vi "4. Event-Driven State Machine - Traffic Light Simulator.vi"() -> ()   [LabVIEW 2018]
uses:
  Typedefs/States for Event-Driven State Machine.ctl
panel:
  in  "stop":bool
  in  "Press Green":bool
  in  "Press Yellow":bool
  in  "Press Red":bool
  out "Yellow":bool
  out "Green":bool
  out "Red":bool
  out "Traffic Lights Picture":picture
  # "Traffic Light Graphic Vector by Vecteezy\n(https://www.vecteezy.com/free-vector/graphic)"
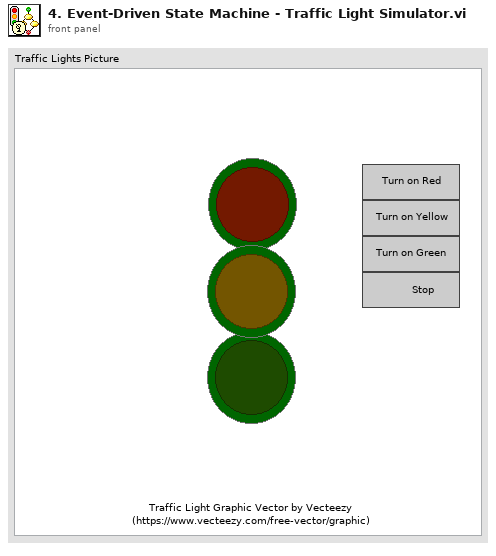
[diagram p1: front panel]
types:
  T1 = typedef "States for Event-Driven State Machine.ctl" = enum16{"Initialize", "Red", "Yellow", "Green", "Wait for Event", "Stop"}
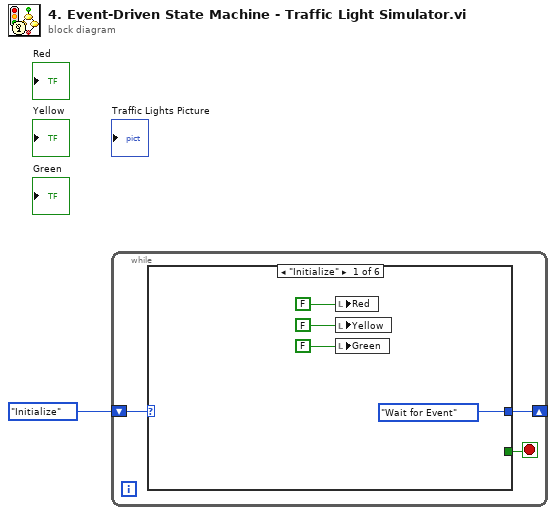
[diagram p0: block diagram]
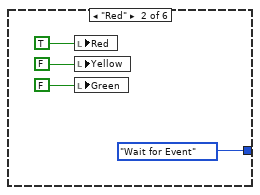
[diagram p2: hidden frame]
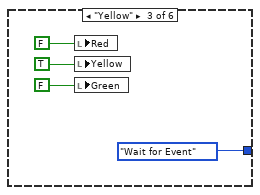
[diagram p3: hidden frame]
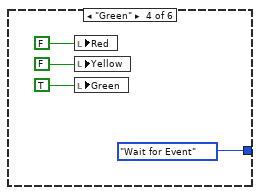
[diagram p4: hidden frame]
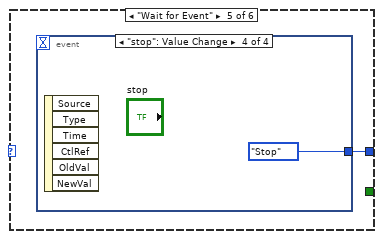
[diagram p5: hidden frame]
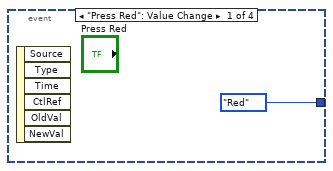
[diagram p6: hidden frame]
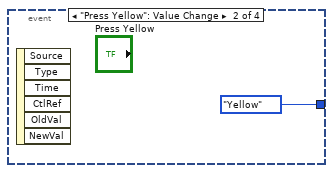
[diagram p7: hidden frame]
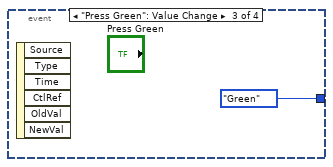
[diagram p8: hidden frame]
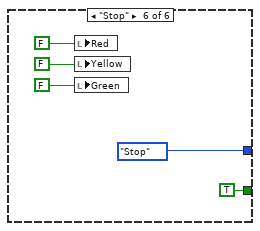
[diagram p9: hidden frame]
diagram:
  n1 = while {
    shift-right: [w3] -> _
    shift-left: States_for_Event-Driven_State_Machine."Initialize" -> [w4]
    stop <- w2 stop-if-true
    n2 = case shown="\"Initialize\"" w4 {
      tunnel: [States_for_Event-Driven_State_Machine."Wait for Event" States_for_Event-Driven_State_Machine."Wait for Event" States_for_Event-Driven_State_Machine."Wait for Event" States_for_Event-Driven_State_Machine."Wait for Event" w21 States_for_Event-Driven_State_Machine."Stop"] -> w3
      tunnel: [_ _ _ _ _ TRUE] -> w2
      frame "Initialize" {
        n3 = local write "Red"(FALSE ("Red")) -> ()
        n4 = local write "Yellow"(FALSE ("Red")) -> ()
        n5 = local write "Green"(FALSE ("Red")) -> ()
      }
      frame "Red" {
        n6 = local write "Red"(TRUE ("Red")) -> ()
        n7 = local write "Yellow"(FALSE ("Red")) -> ()
        n8 = local write "Green"(FALSE ("Red")) -> ()
      }
      frame "Yellow" {
        n9 = local write "Red"(FALSE ("Red")) -> ()
        n10 = local write "Yellow"(TRUE ("Red")) -> ()
        n11 = local write "Green"(FALSE ("Red")) -> ()
      }
      frame "Green" {
        n12 = local write "Red"(FALSE ("Red")) -> ()
        n13 = local write "Yellow"(FALSE ("Red")) -> ()
        n14 = local write "Green"(TRUE ("Red")) -> ()
      }
      frame "Wait for Event" {
        n15 = event shown="[3] \"stop\": Value Change" {
          selector: _ -> [_ _ _ _]
          dyn-events: _ -> [_ _ _ _]
          timeout: _ -> [_ _ _ _]
          tunnel: [States_for_Event-Driven_State_Machine."Red" States_for_Event-Driven_State_Machine."Yellow" States_for_Event-Driven_State_Machine."Green" States_for_Event-Driven_State_Machine."Stop"] -> w21
          event "Press Red": Value Change {
            n16 = event-data() -> ()  [unwired: 1 in, 6 out]
          }
          event "Press Yellow": Value Change {
            n17 = event-data() -> ()  [unwired: 1 in, 6 out]
          }
          event "Press Green": Value Change {
            n18 = event-data() -> ()  [unwired: 1 in, 6 out]
          }
          event "stop": Value Change {
            n19 = event-data() -> ()  [unwired: 1 in, 6 out]
          }
        }
      }
      frame "Stop" {
        n20 = local write "Red"(FALSE ("Red")) -> ()
        n21 = local write "Yellow"(FALSE ("Red")) -> ()
        n22 = local write "Green"(FALSE ("Red")) -> ()
      }
    }
  }
